vi "Define_Stop_Point_for_Bad_101_Subtrack-1.vi"(1 "[IN] Indexes for Jumps":i32[](array[numeric]), 2 "[IN] Dot Statuses":i16[][](array[numeric]), 3 "[IN] Index of Mer\nging (\"101\") Point":i32, 4 "[IN] Current index":i32) -> (0 "[OUT] Continue saving points":bool)   [LabVIEW 2013]
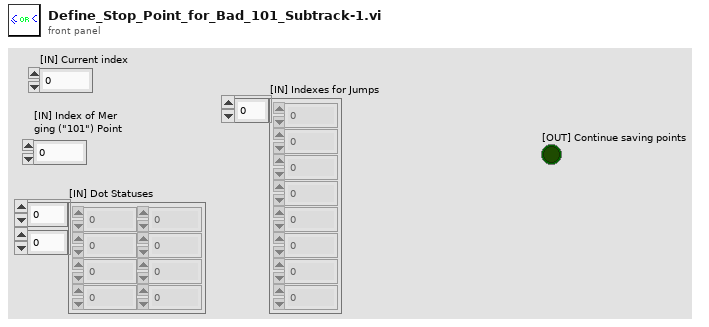
[diagram p1: front panel]
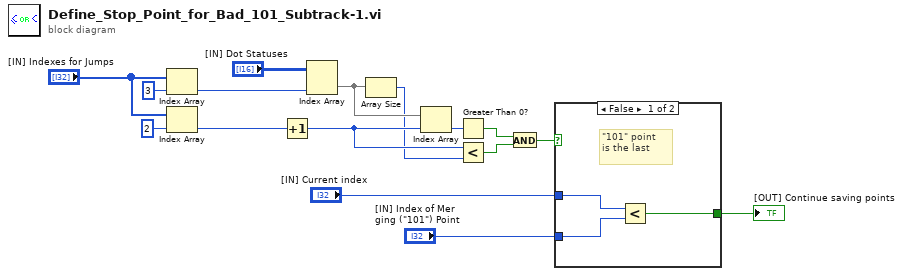
[diagram p0: block diagram]
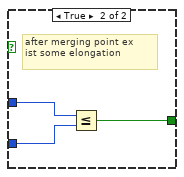
[diagram p2: hidden frame]
diagram:
  n1 = Index Array(array="[IN] Indexes for Jumps", index=3) -> (element=w12:i32)
  n2 = Index Array(array="[IN] Indexes for Jumps", index=2) -> (element=w9:i32)
  n3 = Increment(x=w9) -> (x+1=w8:i32)
  n4 = Index Array(array="[IN] Dot Statuses", index (col)=w12) -> (element=w10:i16[])  [unwired: 1 in]
  n5 = Array Size(array=w10) -> (size(s)=w7:i32)
  n6 = Index Array(array=w10, index=w8) -> (element=w11:i16)
  n7 = Greater Than 0?(x=w11) -> (x > 0?=w6:bool)
  n8 = Less?(x=w8, y=w7) -> (x < y?=w5:bool)
  n9 = And(x=w6, y=w5) -> (x .and. y?=w4:bool)
  n10 = case shown="False" w4 {
    tunnel: "[IN] Current index" -> [w19 w22]
    tunnel: "[IN] Index of Mer\nging (\"101\") Point" -> [w18 w21]
    tunnel: [w17 w20] -> w1
    frame False {
      # "\"101\" point \nis the last"
      n11 = Less?(x=w19, y=w18) -> (x < y?=w17:bool)
    }
    frame True {
      # "after merging point ex\nist some elongation"
      n12 = Less Or Equal?(x=w22, y=w21) -> (x <= y?=w20:bool)
    }
  }
  "[OUT] Continue saving points" <- w1
